vi "OFDM-SIM信号提取.vi"(2 "error in":errorcluster, 3 "M-QAM":i32=4 caption="M-QAM (16)", 4 "待解调信号":cdb[](array[numeric])) -> (0 "error out":errorcluster, 1 "解调信号":i32[](array[numeric]))   [LabVIEW 2018]
uses:
  <vilib>/addons/Modulation/Digital/General/MT Generate QAM System Parameters(M).vi
  <vilib>/addons/Modulation/Digital/General/MT Map QAM Symbols to Bits.vi
  <vilib>/addons/Modulation/niDMT.lvlib
panel:
  out "均衡后的星座图":cdb[](graph)
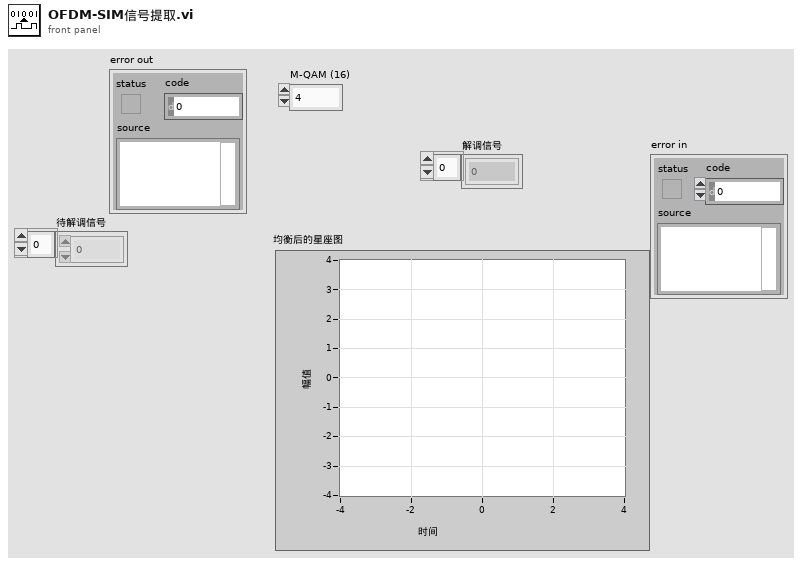
[diagram p1: front panel]
types:
  T1 = cluster{"samples per symbol (16)":i32, "symbol map":cdb[]}
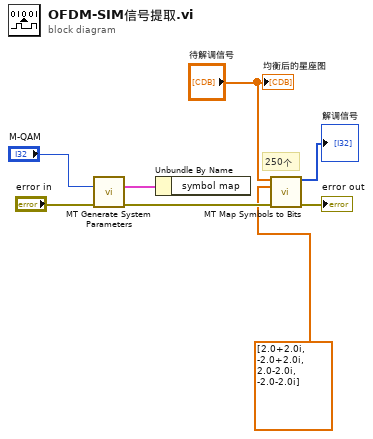
[diagram p0: block diagram]
diagram:
  # "250个"
  n1 = call-poly <vilib>:"MT Generate System Parameters.vi"("M-QAM (16)"="M-QAM", "error in (no error)"="error in") -> ("QAM system parameters"=w8:T1, "error out"=w6:errorcluster)  [unwired: 11 in, 1 out]
  n2 = Unbundle By Name(w8) -> ()  [unwired: 1 out]
  n3 = call-poly <vilib>:"MT Map Symbols to Bits.vi"("symbols"="待解调信号", "symbol map"=cdb[] [2.0+2.0i, -2.0+2.0i, 2.0-2.0i, -2.0-2.0i], "error in (no error)"=w6) -> ("output bit stream"=→"解调信号":i8[], "error out"=→"error out":errorcluster)  [unwired: 11 in]
  "均衡后的星座图" <- "待解调信号"
